vi "notes-in-scale.vi"(11 "Cluster":T1) -> (2 "Array":string[](array[string]), 3 "String":string)   [LabVIEW 2019]
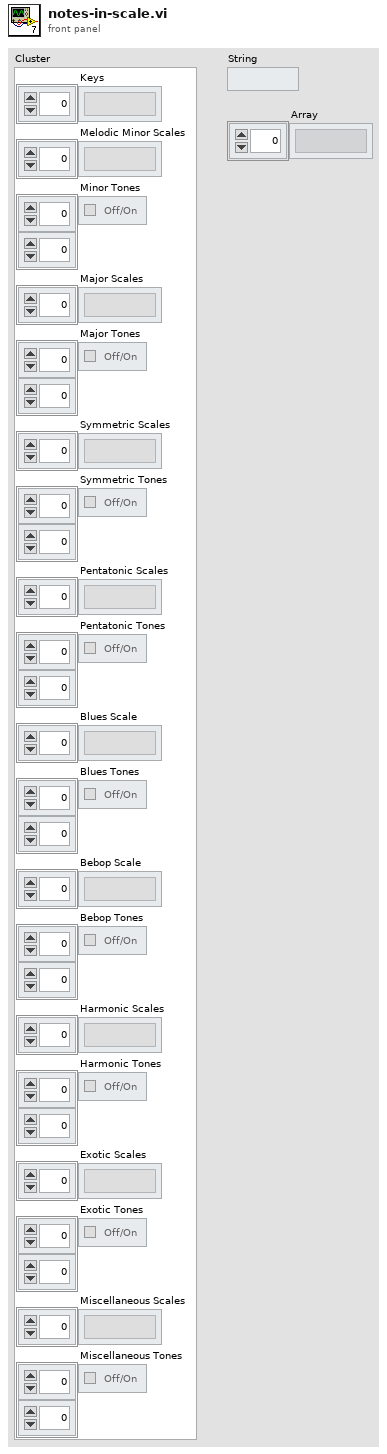
[diagram p1: front panel]
types:
  T1 = cluster{"Keys":string[], "Melodic Minor Scales":string[], "Minor Tones":bool[][], "Major Scales":string[], "Major Tones":bool[][], "Symmetric Scales":string[], "Symmetric Tones":bool[][], "Pentatonic Scales":string[], "Pentatonic Tones":bool[][], "Blues Scale":string[], "Blues Tones":bool[][], "Bebop Scale":string[], "Bebop Tones":bool[][], "Harmonic Scales":string[], "Harmonic Tones":bool[][], "Exotic Scales":string[], "Exotic Tones":bool[][], "Miscellaneous Scales":string[], "Miscellaneous Tones":bool[][]}
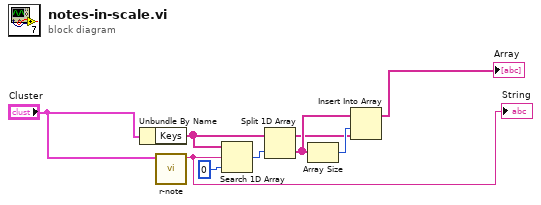
[diagram p0: block diagram]
diagram:
  n1 = Unbundle By Name("Cluster") -> ("Keys"=w9:string[])
  n2 = call "r-note.vi"("Cluster"="Cluster") -> ("String"=w7:string)  [unwired: 10 in]
  "String" <- w7
  n3 = Search 1D Array(1D array=w9, element=w7, start index (0)=0) -> (index of element=w3:i32)
  n4 = Split 1D Array(array=w9, index=w3) -> (first subarray=w4:string[], second subarray=w6:string[])
  n5 = Array Size(array=w6) -> (size(s)=w5:i32)
  n6 = Insert Into Array(array=w6, index=w5, new element=w4) -> (→"Array":string[])
